vi "Updater Convert TDMS File 5.0 to 5.1 PIM.vi"(7 "TDMS Path In":path, 8 "error in (no error)":errorcluster, 11 "TDMS File Ref":refnum<k34>) -> (0 "error out":errorcluster, 3 "TDMS File Ref":refnum<k34>, 5 "TDMS Path Out":path)   [LabVIEW 2011]
uses:
  OpenG.LIB/file/file.llb/Strip Path - Traditional__ogtk.vi
  OpenG.LIB/file/file.llb/Build Path - Traditional__ogtk.vi
  OpenG.LIB/file/file.llb/Convert File Extension (Path)__ogtk.vi
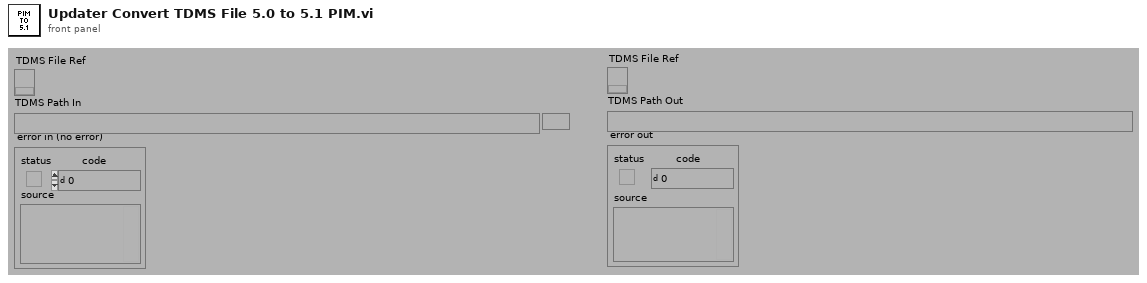
[diagram p1: front panel]
types:
  T1 = enum16{"open", "open or create", "create or replace", "create", "open (read-only)"}
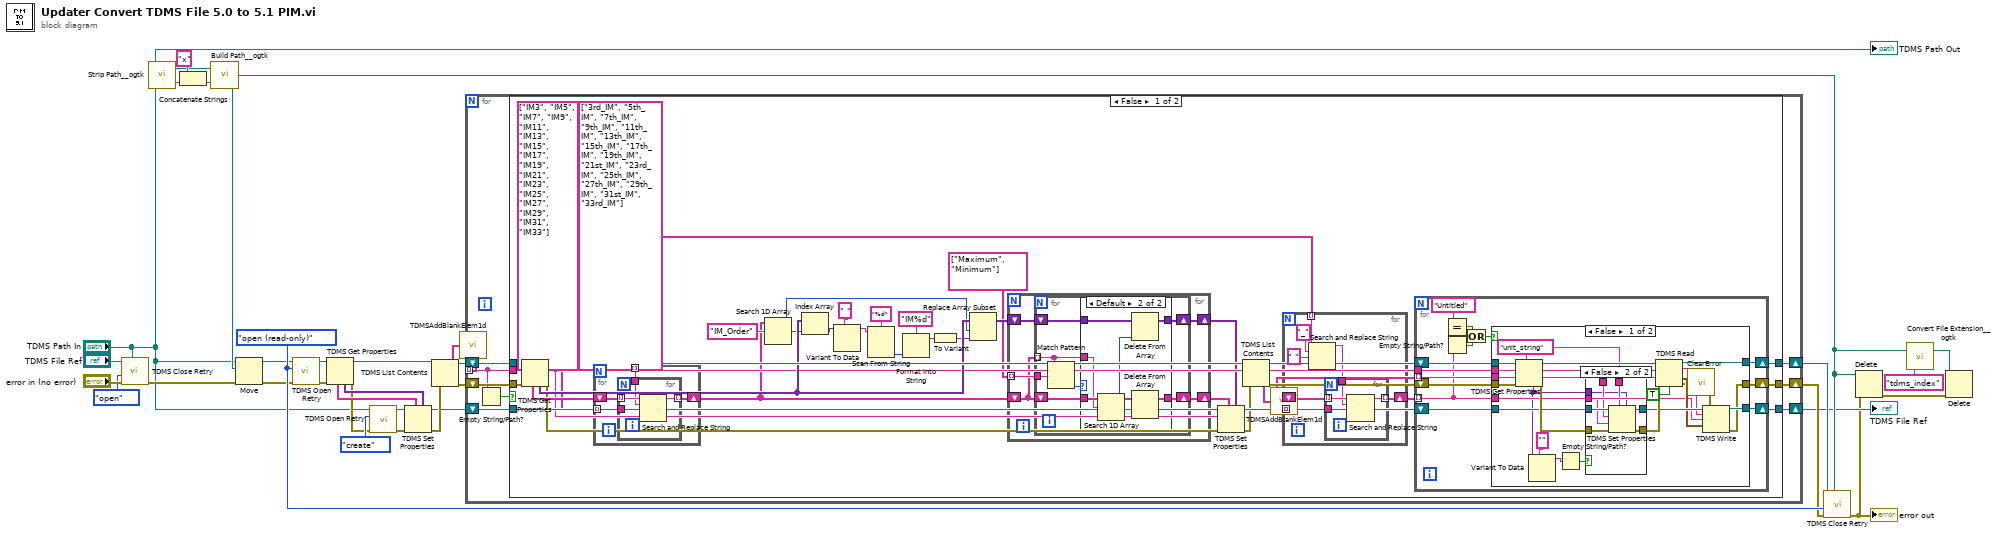
[diagram p0: block diagram]
diagram:
  w34 = T1."open (read-only)" ("operation (0:open)")
  n1 = call "TDMS Close Retry.vi"("TDMS Path"="TDMS Path In", "error in (no error)"="error in (no error)", "Operation (0:open)"=T1."open" ("operation (0:open)"), "TDMS File Ref"="TDMS File Ref") -> ("error out"=w10:errorcluster)  [unwired: 1 in, 6 out]
  n2 = call-poly "Strip Path__ogtk.vi"("path"="TDMS Path In") -> ("stripped path"=w3:path, "name"=w4:string)
  n3 = Concatenate Strings("x" ("string"), w4) -> (w16:string)
  n4 = call-poly "Build Path__ogtk.vi"("name or relative path"=w16, "base path"=w3) -> ("appended path"=w12:path)
  n5 = Move(source path="TDMS Path In", error in=w10, 10:w12) -> (error out=w18:errorcluster, 3:w17:path)  [unwired: 3 out]
  n6 = call "TDMS Open Retry.vi"("error in (no error)"=w18, "Operation (0:open)"=w34, "Path"=w17) -> ("error out"=w27:errorcluster, "TDMS File Ref"=w33:refnum<k34>)  [unwired: 1 in, 6 out]
  n7 = TDMS Get Properties(8:w27, 11:w33) -> (0:w13:errorcluster, 3:w29:refnum<k34>, 4:w14:variant[], 6:w15:string[])  [unwired: 1 in, 5 out]
  n8 = call "TDMS Open Retry.vi"("error in (no error)"=w13, "Operation (0:open)"=T1."create" ("operation (0:open)"), "Path"="TDMS Path In") -> ("error out"=w26:errorcluster, "TDMS File Ref"=w25:refnum<k34>)  [unwired: 1 in, 6 out]
  n9 = TDMS Set Properties(5:w14, 7:w15, 8:w26, 11:w25) -> (0:w32:errorcluster, 3:w24:refnum<k34>)  [unwired: 4 out]
  n10 = TDMS List Contents(4:w32, 7:w29) -> (0:w31:errorcluster, 2:w1:string[], 3:w23:refnum<k34>)  [unwired: 2 out]
  n11 = call <vilib>:"TDMSAddBlankElem1d.vi"("input string array"=w1) -> ("output string array with blank element at the beginning"=w35:string[])
  n12 = for {
    shift-right: [w41] -> w30
    shift-left: w31 -> [w42]
    tunnel: w35 -> [w40] mode=indexing
    shift-right: [w37] -> w22
    shift-left: w23 -> [w43]
    shift-right: [w36] -> w7
    shift-left: w24 -> [w39]
    n13 = Empty String/Path?(string/path=w40) -> (empty?=w38:bool)
    n14 = case shown="False" w38 {
      tunnel: w43 -> [w80 w172]
      tunnel: w42 -> [w79 w173]
      tunnel: [w72 w173] -> w41
      tunnel: w40 -> [w78 _]
      tunnel: w39 -> [w64 w171]
      tunnel: [w75 w172] -> w37
      tunnel: [w74 w171] -> w36
      frame False {
        w70 = string[] ["3rd_IM", "5th_IM", "7th_IM", "9th_IM", "11th_IM", "13th_IM", "15th_IM", "17th_IM", "19th_IM", "21st_IM", "23rd_IM", "25th_IM", "27th_IM", "29th_IM", "31st_IM", "33rd_IM"]
        w61 = string[] ["IM3", "IM5", "IM7", "IM9", "IM11", "IM13", "IM15", "IM17", "IM19", "IM21", "IM23", "IM25", "IM27", "IM29", "IM31", "IM33"]
        n15 = TDMS Get Properties(8:w79, 10:w78, 11:w80) -> (0:w60:errorcluster, 2:w62:string, 3:w77:refnum<k34>, 4:w67:variant[], 6:w66:string[])  [unwired: 1 in, 3 out]
        n16 = for {
          tunnel: w70 -> [w113] mode=indexing
          tunnel: w61 -> [w112] mode=indexing
          shift-right: [w114] -> w48
          shift-left: w66 -> [w115]
          n17 = for {
            tunnel: w115 -> [w119] mode=indexing
            tunnel: [w118] -> w114 mode=indexing
            tunnel: w113 -> [w117]
            tunnel: w112 -> [w116]
            n18 = Search and Replace String(input string=w119, search string=w117, replace string=w116) -> (result string=w118:string)  [unwired: 2 in, 6 out]
          }
        }
        n19 = Search 1D Array(1D array=w48, element="IM_Order") -> (index of element=w50:i32)  [unwired: 1 out]
        n20 = Index Array(array=w67, index=w50) -> (element=w58:variant)
        n21 = Variant To Data(type=" " ("replace string (\"\")"), Variant=w58) -> (data=w54:string)  [unwired: 1 in, 1 out]
        n22 = Scan From String(format string="%d", input string=w54) -> (output 1=w53:i32)  [unwired: 2 in, 4 out]
        n23 = Format Into String(format string="IM%d", w53) -> (resulting string=w52:string)  [unwired: 2 in, 1 out]
        n24 = To Variant(anything=w52) -> (Variant=w51:variant)
        n25 = Replace Array Subset(array=w67, new element=w51, index=w50) -> (w49:variant[])
        n26 = for {
          shift-right: [w84] -> w46
          shift-left: w48 -> [w81]
          shift-right: [w83] -> w45
          shift-left: w49 -> [w85]
          tunnel: string[] ["Maximum", "Minimum"] ("second subarray 2") -> [w82] mode=indexing
          n27 = for {
            shift-right: [w89] -> w83
            shift-left: w85 -> [w92]
            shift-right: [w90] -> w84
            shift-left: w81 -> [w91]
            tunnel: w82 -> [w88]
            tunnel: w81 -> [w86] mode=indexing
            n28 = Match Pattern(string=w86, regular expression=w88) -> (offset past match=w87:i32)  [unwired: 4 out]
            n29 = case shown="Default" w87 {
              tunnel: w92 -> [w94 w100]
              tunnel: w91 -> [w93 w99]
              tunnel: [w93 w97] -> w90
              tunnel: [w94 w96] -> w89
              tunnel: w86 -> [_ w95]
              frame -1 {
              }
              frame Default {
                n30 = Search 1D Array(1D array=w99, element=w95) -> (index of element=w98:i32)  [unwired: 1 out]
                n31 = Delete From Array(array=w100, index=w98) -> (array with subset deleted=w96:variant[])  [unwired: 1 in, 1 out]
                n32 = Delete From Array(array=w99, index=w98) -> (array with subset deleted=w97:string[])  [unwired: 1 in, 1 out]
              }
            }
          }
        }
        n33 = TDMS Set Properties(5:w45, 7:w46, 8:w60, 10:w62, 11:w64) -> (0:w63:errorcluster, 3:w65:refnum<k34>)  [unwired: 3 out]
        n34 = TDMS List Contents(4:w63, 6:w62, 7:w77) -> (0:w73:errorcluster, 1:w44:string[], 2:w71:string, 3:w76:refnum<k34>)
        n35 = call <vilib>:"TDMSAddBlankElem1d.vi"("input string array"=w44) -> ("output string array with blank element at the beginning"=w69:string[])
        n36 = for {
          tunnel: w70 -> [w104] mode=indexing
          tunnel: w61 -> [w105] mode=indexing
          shift-right: [w106] -> w68
          shift-left: w69 -> [w107]
          n37 = Search and Replace String(input string=w104, search string="_", replace string=" " ("replace string (\"\")")) -> (result string=w101:string)  [unwired: 1 in, 7 out]
          n38 = for {
            tunnel: w107 -> [w111] mode=indexing
            tunnel: [w110] -> w106 mode=indexing
            tunnel: w101 -> [w109]
            tunnel: w105 -> [w108]
            n39 = Search and Replace String(input string=w111, search string=w109, replace string=w108) -> (result string=w110:string)  [unwired: 2 in, 6 out]
          }
        }
        n40 = for {
          shift-right: [w125] -> w75
          shift-left: w76 -> [w130]
          shift-right: [w127] -> w74
          shift-left: w65 -> [w132]
          shift-right: [w126] -> w72
          shift-left: w73 -> [w131]
          tunnel: w71 -> [w129]
          tunnel: w69 -> [w128] mode=indexing
          tunnel: w68 -> [w124] mode=indexing
          n41 = Equal?(x="Untitled" ("string"), y=w124) -> (x = y?=w121:bool)
          n42 = Empty String/Path?(string/path=w124) -> (empty?=w122:bool)
          n43 = Or(x=w121, y=w122) -> (x .or. y?=w120:bool)
          n44 = case shown="False" w120 {
            tunnel: w132 -> [w156 w169]
            tunnel: w131 -> [w155 w168]
            tunnel: w130 -> [w154 w170]
            tunnel: w129 -> [w153 _]
            tunnel: w128 -> [w152 _]
            tunnel: [w144 w169] -> w127
            tunnel: [w143 w168] -> w126
            tunnel: [w142 w170] -> w125
            tunnel: w124 -> [w139 _]
            frame False {
              w141 = "unit_string" ("string")
              n45 = TDMS Get Properties(7:w141, 8:w155, 9:w152, 10:w153, 11:w154) -> (0:w157:errorcluster, 1:w140:string, 2:w148:string, 3:w151:refnum<k34>, 4:w136:variant)  [unwired: 2 out]
              n46 = Variant To Data(type="" ("element"), Variant=w136) -> (data=w138:string)  [unwired: 1 in, 1 out]
              n47 = Empty String/Path?(string/path=w138) -> (empty?=w135:bool)
              n48 = case shown="False" w135 {
                tunnel: w157 -> [w158 w167]
                tunnel: w156 -> [w159 w166]
                tunnel: [w158 w165] -> w150
                tunnel: w148 -> [_ w164]
                tunnel: [w159 w163] -> w147
                tunnel: w141 -> [_ w162]
                tunnel: w139 -> [_ w161]
                tunnel: w136 -> [_ w160]
                frame True {
                }
                frame False {
                  n49 = TDMS Set Properties(5:w160, 7:w162, 8:w167, 9:w161, 10:w164, 11:w166) -> (0:w165:errorcluster, 3:w163:refnum<k34>)  [unwired: 2 out]
                }
              }
              n50 = TDMS Read(0:w151, 5:w148, 7:w140, 11:w150, 13:TRUE ("return channels in file order? (F)")) -> (4:w142:refnum<k34>, 6:w145:string, 10:w146:waveform(dbl), 15:w134:errorcluster)  [unwired: 3 in, 2 out]
              n51 = call <vilib>:"ClearError.vi"("error in (no error)"=w134) -> ("error out"=w149:errorcluster)
              n52 = TDMS Write(0:w147, 5:w145, 7:w139, 9:w146, 11:w149) -> (4:w144:refnum<k34>, 15:w143:errorcluster)  [unwired: 1 in, 2 out]
            }
            frame True {
            }
          }
        }
      }
      frame True {
      }
    }
  }
  "TDMS File Ref" <- w7
  n53 = call "TDMS Close Retry.vi"("TDMS Path"=w12, "error in (no error)"=w30, "Operation (0:open)"=w34, "TDMS File Ref"=w22) -> ("error out"=w6:errorcluster)  [unwired: 1 in, 6 out]
  "error out" <- w6
  n54 = Delete(path (use dialog)=w12, error in=w6) -> (error out=w21:errorcluster)  [unwired: 5 out]
  n55 = call-poly "Convert File Extension__ogtk.vi"("new ending (none)"="tdms_index", "file name"=w12) -> ("new filename"=w20:path)  [unwired: 1 out]
  n56 = Delete(path (use dialog)=w20, error in=w21) -> ()  [unwired: 6 out]
  "TDMS Path Out" <- "TDMS Path In"
